vi "Add Waveform Sections.vi"(8 "error in":errorcluster, 10 "Wfm Pointers":T1[](array[typedef]), 11 "CustomDevice Ref":T2 format="%.0x") -> (0 "error out":errorcluster, 3 "CustomDevice Ref":T2 format="%.0x")   [LabVIEW 2020, in "Waveform-Processing-Custom-Device System Explorer.lvlib"]
uses:
  Waveform-Processing-Custom-Device System Explorer.lvlib
  <vilib>/NI VeriStand/Custom Device API/Custom Device Item Ref.ctl
  <vilib>/NI VeriStand/Custom Device API/Custom Device Pointer.ctl
  NationalInstruments.VeriStand.SystemStorage
  NationalInstruments.VeriStand
  Shared/Constants.vi
  <vilib>/NI VeriStand/Custom Device API/Set Item Property (Dependent Node Pointer).vi
  <vilib>/NI VeriStand/Custom Device API/Custom Device API.lvlib
  Shared/Waveform-Processing-Custom-Device Shared.lvlib
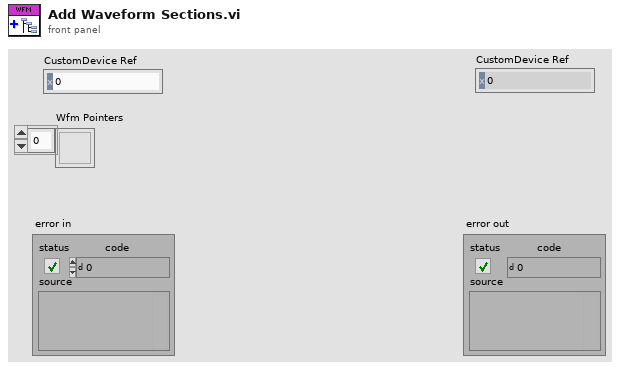
[diagram p1: front panel]
types:
  T1 = typedef "Custom Device API.lvlib/Custom Device Pointer.ctl" = refnum<k24>
  T2 = typedef "Custom Device API.lvlib/Custom Device Item Ref.ctl" = u64
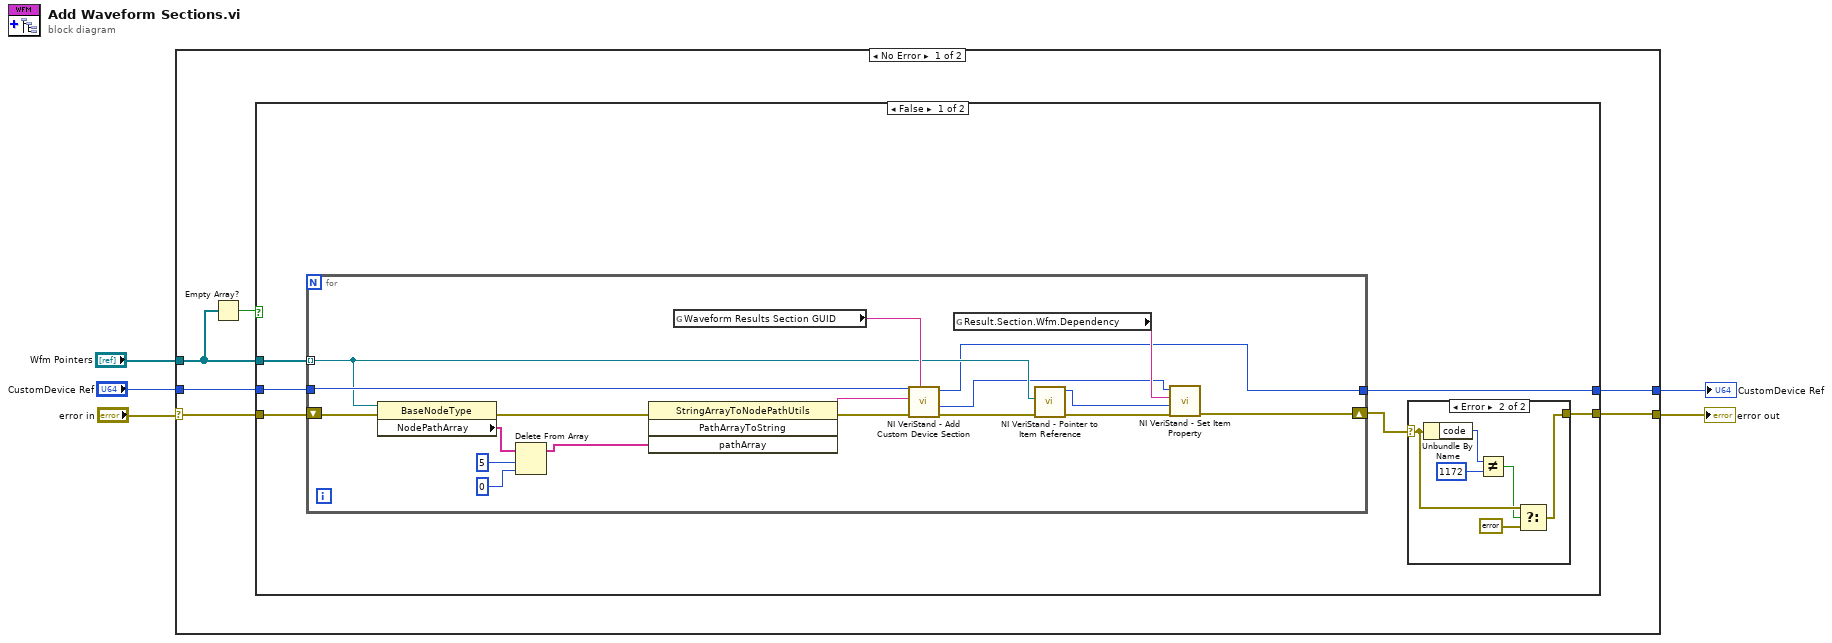
[diagram p0: block diagram]
diagram:
  n1 = case shown="No Error" "error in" {
    selector: "error in" -> [w10 w46]
    tunnel: [w9 w46] -> w4
    tunnel: "CustomDevice Ref" -> [w11 w45]
    tunnel: [w8 w45] -> w2
    tunnel: "Wfm Pointers" -> [w7 _]
    frame No Error {
      n2 = Empty Array?(array=w7) -> (empty?=w6:bool)
      n3 = case shown="False" w6 {
        tunnel: w7 -> [w17 _]
        tunnel: w11 -> [w16 w44]
        tunnel: w10 -> [w15 w43]
        tunnel: [w12 w43] -> w9
        tunnel: [w14 w44] -> w8
        frame False {
          n4 = for {
            tunnel: w16 -> [w42]
            tunnel: w17 -> [w36] mode=indexing
            tunnel: [w32] -> w14
            shift-right: [w33] -> w13
            shift-left: w15 -> [w40]
            n5 = property class="BaseNodeType"(reference=w36, error in=w40) -> (error out=w31:errorcluster, "NodePathArray"=w27:string[])  [unwired: 1 out]
            n6 = Delete From Array(array=w27, length=5, index=0) -> (array with subset deleted=w25:string[])  [unwired: 1 out]
            n7 = invoke class="StringArrayToNodePathUtils" method="PathArrayToString"(error in=w31, "pathArray"=w25) -> (error out=w30:errorcluster, "PathArrayToString"=w26:string)  [unwired: 2 in, 2 out]
            n8 = global read "Constants.vi" "Waveform Results Section GUID"() -> (w41:string)
            n9 = call <vilib>:"NI VeriStand - Add Custom Device Section.vi"("GUID (Default Section)"=w41, "error in (no error)"=w30, "Section Name"=w26, "Parent Ref in"=w42) -> ("error out"=w38:errorcluster, "Section Ptr"=w34:T2, "Parent Ref out"=w32:T2)  [unwired: 4 in, 1 out]
            n10 = global read "Constants.vi" "Result.Section.Wfm.Dependency"() -> (w39:string)
            n11 = call <vilib>:"NI VeriStand - Pointer to Item Reference.vi"("error in (no error)"=w38, "Node Pointer"=w36) -> ("error out"=w37:errorcluster, "Item Ref out"=w35:T2)  [unwired: 8 in]
            n12 = call-poly <vilib>:"NI VeriStand - Set Item Property.vi"("error in (no error)"=w37, "Dependent Node Ref"=w35, "Property Name"=w39, "Item Ref in"=w34) -> ("error out"=w33:errorcluster)  [unwired: 5 in, 2 out]
          }
          n13 = case shown="Error" w13 {
            selector: w13 -> [w18 w22]
            tunnel: [w18 w19] -> w12
            frame No Error {
            }
            frame Error {
              n14 = Unbundle By Name(w22) -> ("code"=w24:i32)
              n15 = Not Equal?(x=w24, y=1172) -> (x != y?=w21:bool)
              n16 = Select(t=w22, s=w21, f=errorcluster {"status"=FALSE, "code"=0, "source"=""}) -> (s? t:f=w19:errorcluster)
            }
          }
        }
        frame True {
        }
      }
    }
    frame Error {
    }
  }
  "error out" <- w4
  "CustomDevice Ref" <- w2
